vi "Find Help Documentation in Project.vi"(8 "error in (no error)":errorcluster, 11 "Project Path":path) -> (0 "error out":errorcluster, 1 "Main Page":string, 2 "Support":string[](array[string]), 3 "Other Pages":string[](array[string]), 4 "Help Documentation Path":path)   [LabVIEW 2015, in "HTML Help File Tools.lvlib"]
uses:
  HTML Help File Tools.lvlib
  Log FGV Operation Modes.ctl
  Error Location.ctl
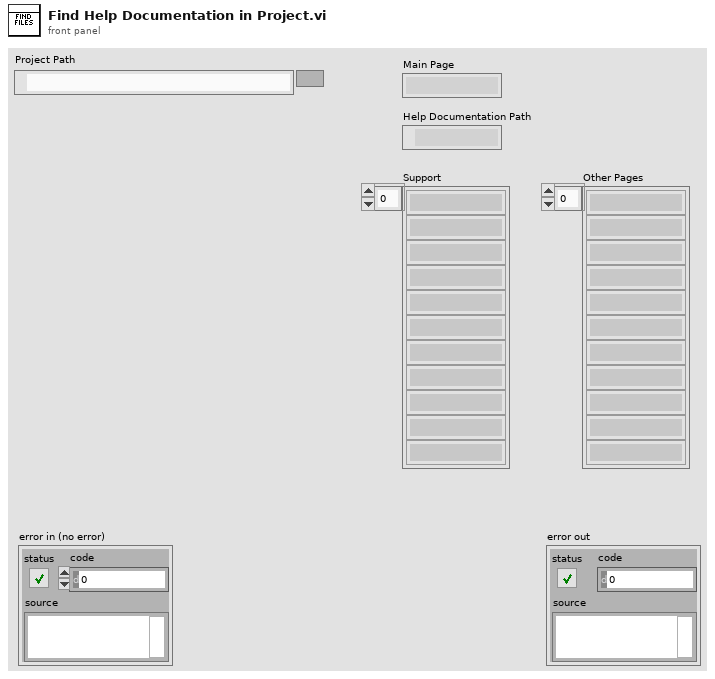
[diagram p1: front panel]
types:
  T1 = typedef "HTML Help File Tools.lvlib/Error Location.ctl" = enum16{"Delete tmp", "Compile HHP", "Find Install", "Create tmp", "Create HHP", "Find Help"}
  T2 = typedef "HTML Help File Tools.lvlib/Log FGV Operation Modes.ctl" = enum16{"Close", "Write", "Open File"}
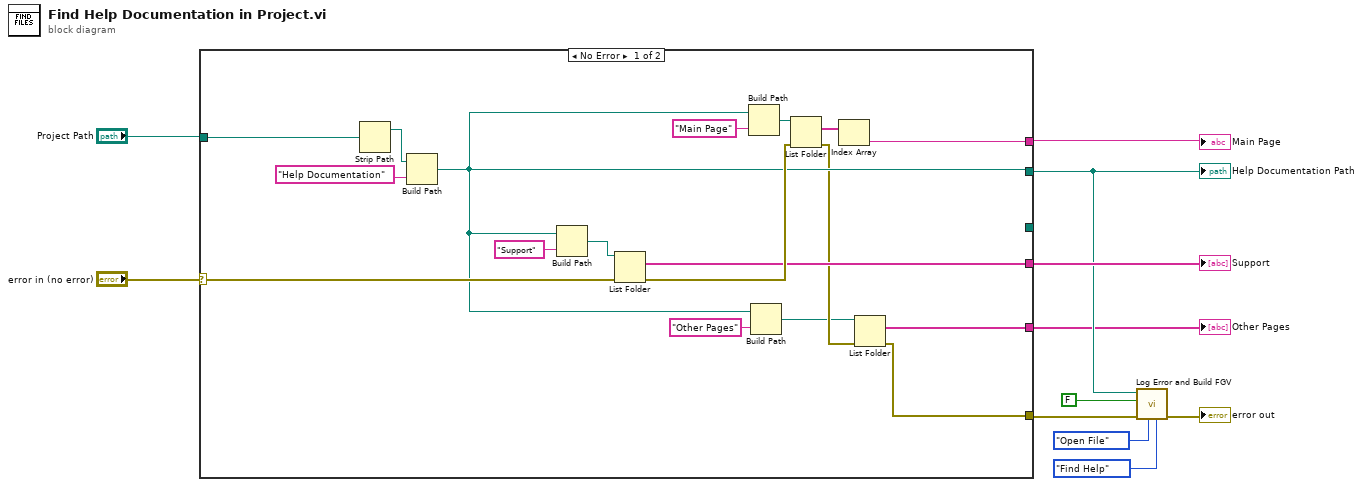
[diagram p0: block diagram]
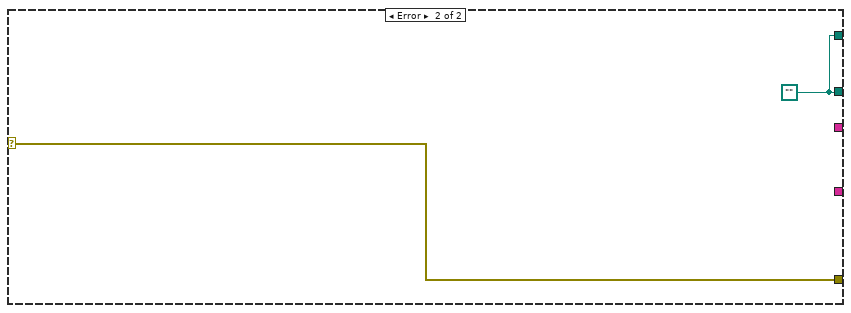
[diagram p2: hidden frame]
diagram:
  n1 = case shown="No Error" "error in (no error)" {
    selector: "error in (no error)" -> [w29 w31]
    tunnel: [w12 w31] -> w7
    tunnel: "Project Path" -> [w20 _]
    tunnel: [w19 _] -> w9
    tunnel: [w18 _] -> w8
    tunnel: [_ w30] -> _
    tunnel: [w17 w30] -> w2
    tunnel: [w13 _] -> w1
    frame No Error {
      n2 = Strip Path(path=w20) -> (stripped path=w22:path)  [unwired: 1 out]
      n3 = Build Path(base path=w22, name or relative path="Help Documentation") -> (appended path=w17:path)
      n4 = Build Path(base path=w17, name or relative path="Support") -> (appended path=w23:path)
      n5 = List Folder(path=w23, error in=w29) -> (filenames=w18:string[], error out=w21:errorcluster)  [unwired: 2 in, 2 out]
      n6 = Build Path(base path=w17, name or relative path="Main Page") -> (appended path=w25:path)
      n7 = Build Path(base path=w17, name or relative path="Other Pages") -> (appended path=w14:path)
      n8 = List Folder(path=w25, error in=w21) -> (filenames=w24:string[], error out=w15:errorcluster)  [unwired: 2 in, 2 out]
      n9 = Index Array(array=w24) -> (element=w19:string)  [unwired: 1 in]
      n10 = List Folder(path=w14, error in=w15) -> (filenames=w13:string[], error out=w12:errorcluster)  [unwired: 2 in, 2 out]
    }
    frame Error {
      w30 = path ""
    }
  }
  "Main Page" <- w9
  "Support" <- w8
  "Help Documentation Path" <- w2
  "Other Pages" <- w1
  n11 = call "Log Error and Build FGV.vi"("Error Location"=Error_Location."Find Help", "Operation Mode"=Log_FGV_Operation_Modes."Open File", "error in"=w7, "Log Build Output?"=FALSE, "Help Documentation Path"=w2) -> ("error out"=→"error out":errorcluster)  [unwired: 6 in]
